vi "LHF.DB.Mongo.Collection.CreateCollection.vi"(8 "error in (no error)":errorcluster, 10 "collectionName":string, 11 "LHF.DB.Mongo in":refnum<class "LHF.DB.Mongo.lvclass">) -> (0 "error out":errorcluster, 3 "LHF.DB.Mongo out":refnum<class "LHF.DB.Mongo.lvclass">)   [LabVIEW 2013, in "LHF.DB.Mongo.lvclass"]
uses:
  LHF.DB.Mongo.lvclass
  LHF.DB.Mongo.lvclass/LHF.DB.Mongo.ctl
  C:/Users/schim/Desktop/Projetos/LabVIEW-MongoDB/src/Driver/MongoDB.Driver.dll
  Driver/MongoDB.Driver.dll
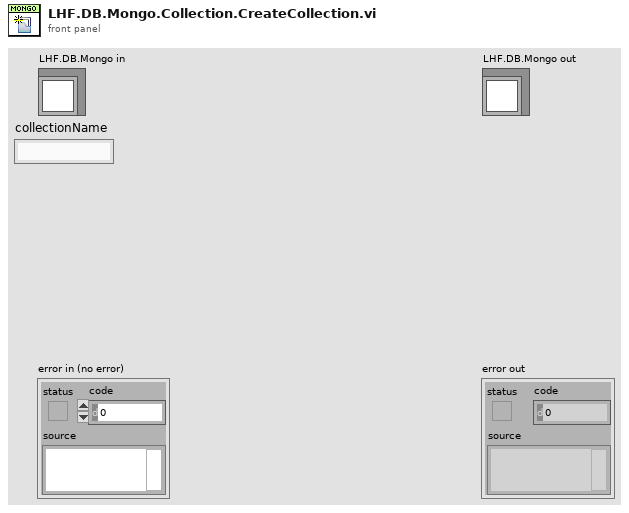
[diagram p1: front panel]
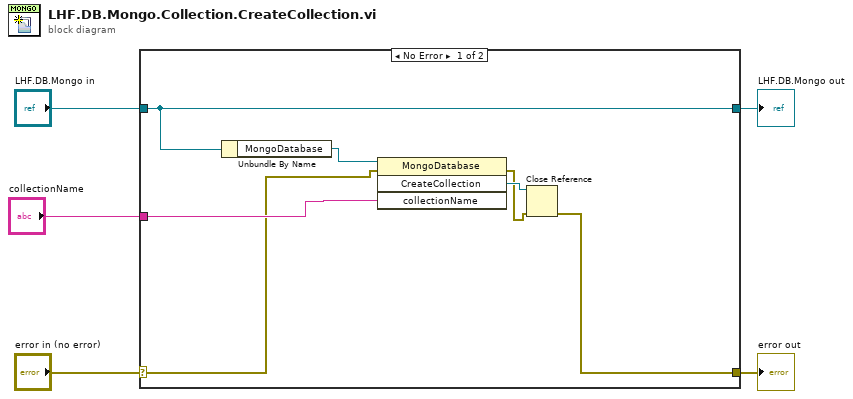
[diagram p0: block diagram]
diagram:
  n1 = case shown="No Error" "error in (no error)" {
    selector: "error in (no error)" -> [w9 w14]
    tunnel: [w6 w14] -> w4
    tunnel: [w12 w13] -> w2
    tunnel: "LHF.DB.Mongo in" -> [w12 w13]
    tunnel: "collectionName" -> [w10 _]
    frame No Error {
      n2 = Unbundle By Name(w12) -> ("MongoDatabase"=w11:refnum<k24>)
      n3 = invoke class="MongoDatabase" method="CreateCollection"(reference=w11, error in=w9, "collectionName"=w10) -> (error out=w7:errorcluster, "CreateCollection"=w8:refnum<k24>)  [unwired: 1 in, 2 out]
      n4 = Close Reference(reference=w8, error in (no error)=w7) -> (error out=w6:errorcluster)
    }
    frame Error {
    }
  }
  "error out" <- w4
  "LHF.DB.Mongo out" <- w2
